vi "waitNotifierStopServer.vi"(8 "error in (no error)":errorcluster, 11 "TcpServerCmd in":refnum<class "TcpServerCmd.lvclass">) -> (0 "error out":errorcluster, 2 "stopServer":bool, 3 "TcpServerCmd out":refnum<class "TcpServerCmd.lvclass">)   [LabVIEW 2018, in "TcpServerCmd.lvclass"]
doc: "Wait to stop the runServer.vi. This is a non-block call function."
uses:
  TcpServerCmd.lvclass
  home/pcortes/Documents/github/ts_labview_tcp_json/src/TcpServerBase/TcpServerBase.lvclass
  TcpServerBase/TcpServerBase.lvclass/TcpServerBase.ctl
  TcpServerBase/TcpServerBase.lvclass
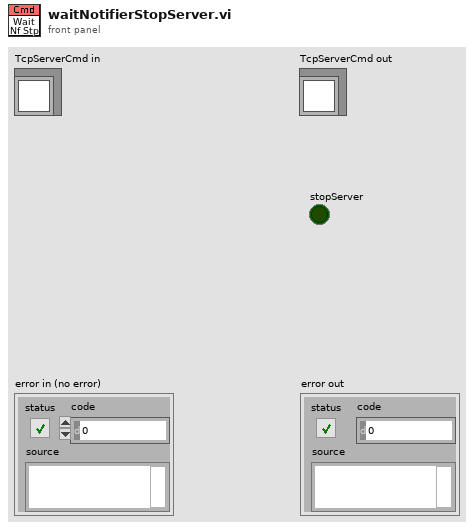
[diagram p1: front panel]
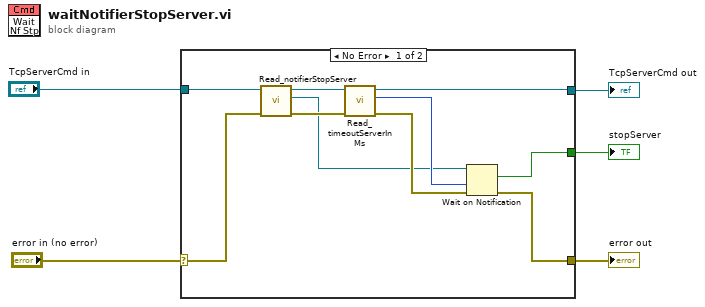
[diagram p0: block diagram]
diagram:
  n1 = case shown="No Error" "error in (no error)" {
    selector: "error in (no error)" -> [w15 w17]
    tunnel: "TcpServerCmd in" -> [w8 w16]
    tunnel: [w11 w17] -> w3
    tunnel: [w14 w16] -> w2
    tunnel: [w10 _] -> w1
    frame No Error {
      n2 = call "Read_notifierStopServer.vi"("error in (no error)"=w15, "TcpServerBase in"=w8) -> ("error out"=w9:errorcluster, "notifierStopServer"=w6:refnum<notifier>, "TcpServerBase out"=w7:refnum<class "TcpServerCmd.lvclass">)  [unwired: 7 in]
      n3 = call "Read_timeoutServerInMs.vi"("error in (no error)"=w9, "TcpServerBase in"=w7) -> ("error out"=w12:errorcluster, "timeoutServerInMs"=w13:i32, "TcpServerBase out"=w14:refnum<class "TcpServerCmd.lvclass">)  [unwired: 7 in]
      n4 = Wait on Notification(notifier=w6, timeout in ms (-1)=w13, error in (no error)=w12) -> (notification=w10:bool, error out=w11:errorcluster)  [unwired: 1 in, 2 out]
    }
    frame Error {
    }
  }
  "error out" <- w3
  "TcpServerCmd out" <- w2
  "stopServer" <- w1
